vi "Problem2.3.vi"() -> ()   [LabVIEW 2019]
panel:
  out "Timer Done":bool
  in  "Wait Time (Seconds)":dbl=4.0
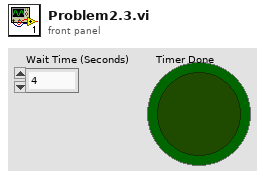
[diagram p1: front panel]
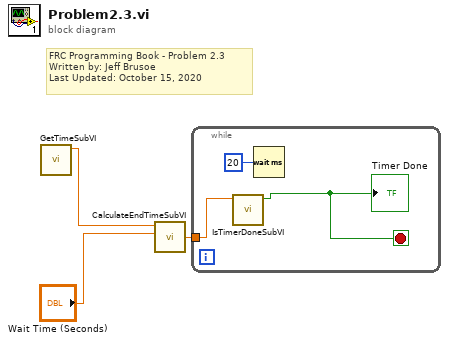
[diagram p0: block diagram]
diagram:
  # "FRC Programming Book - Problem 2.3\nWritten by: Jeff Brusoe\nLast Updated: October 15, 2020"
  n1 = call "GetTimeSubVI.vi"() -> ("Milliseconds"=w1:dbl)  [unwired: 11 in]
  n2 = call "CalculateEndTimeSubVI.vi"("Wait Time (Seconds)"="Wait Time (Seconds)", "Current Time (Seconds)"=w1) -> ("End Time (Seconds)"=w2:dbl)  [unwired: 9 in]
  n3 = while {
    tunnel: w2 -> [w5]
    stop <- w4 stop-if-true
    n4 = call "IsTimerDoneSubVI.vi"("End Time (Seconds)"=w5) -> ("Boolean"=w4:bool)  [unwired: 10 in]
    "Timer Done" <- w4
    n5 = Wait (ms)(milliseconds to wait=u32 20) -> ()  [unwired: 1 out]
  }
